vi "Puntje 6 vertragen.vi"() -> ()   [LabVIEW 2019]
panel:
  in  "Afstand tot voorligger":dbl(slide) scale=0.0..100.0
  out "Wat doet de auto?":string="Auto rijdt gewoon verder"
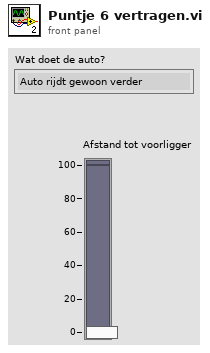
[diagram p1: front panel]
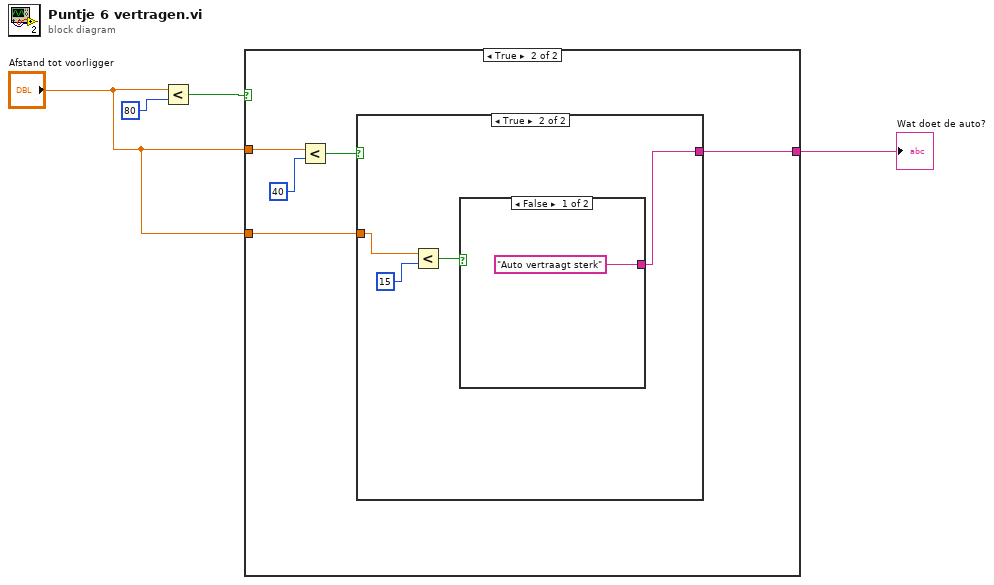
[diagram p0: block diagram]
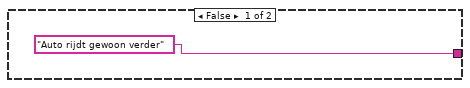
[diagram p2: hidden frame]
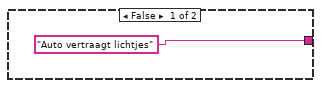
[diagram p3: hidden frame]
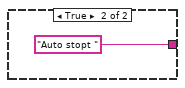
[diagram p4: hidden frame]
diagram:
  n1 = Less?(x="Afstand tot voorligger", y=80) -> (x < y?=w3:bool)
  n2 = case shown="True" w3 {
    tunnel: ["Auto rijdt gewoon verder" w7] -> w2
    tunnel: "Afstand tot voorligger" -> [_ w9]
    tunnel: "Afstand tot voorligger" -> [_ w6]
    frame False {
    }
    frame True {
      n3 = Less?(x=w9, y=40) -> (x < y?=w8:bool)
      n4 = case shown="True" w8 {
        tunnel: ["Auto vertraagt lichtjes" w12] -> w7
        tunnel: w6 -> [_ w15]
        frame False {
        }
        frame True {
          n5 = Less?(x=w15, y=15) -> (x < y?=w13:bool)
          n6 = case shown="False" w13 {
            tunnel: ["Auto vertraagt sterk" "Auto stopt "] -> w12
            frame False {
            }
            frame True {
            }
          }
        }
      }
    }
  }
  "Wat doet de auto?" <- w2
